vi "extract_calibration_standard_point_locations_debug.vi"() -> ()   [LabVIEW 2019]
uses:
  ParametersGlobal.vi
  <vilib>/vision/NI_Vision_Development_Module.lvlib
panel:
  out "Particle Measurements (Pixels)":dbl[][](array[numeric]) format="%.2f"
  out "Camera Input":T1(plugin-control)
  in  "Calibration file in":string="C:\\Users\\Mochi\\Dropbox\\LeiferShaevitz\\Github\\ProjectAPI\\LabviewVIs\\BoxA-PC_projector_to_camera_distortion.png"
  out "error out":errorcluster
  in  "error in (no error)":errorcluster
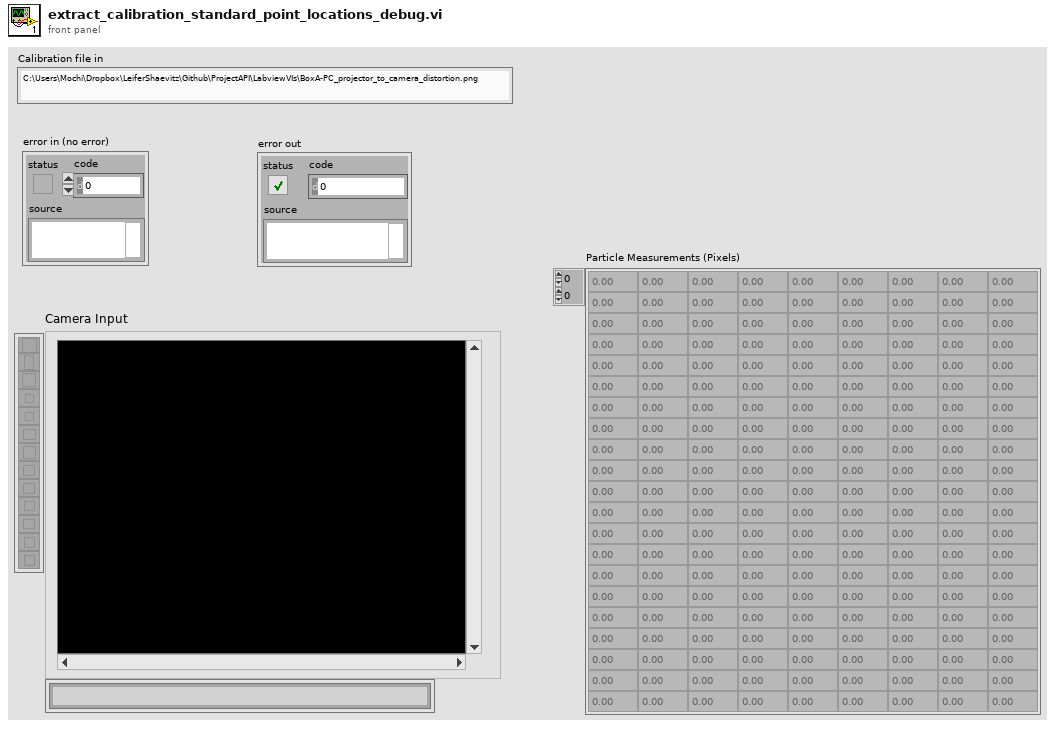
[diagram p1: front panel]
types:
  T1 = typedef "IMAQ Image.ctl" = refnum<image>
  T2 = typedef "Image Type" = u32
  T3 = cluster{"Left":i32, "Top":i32, "Right":i32, "Bottom":i32}
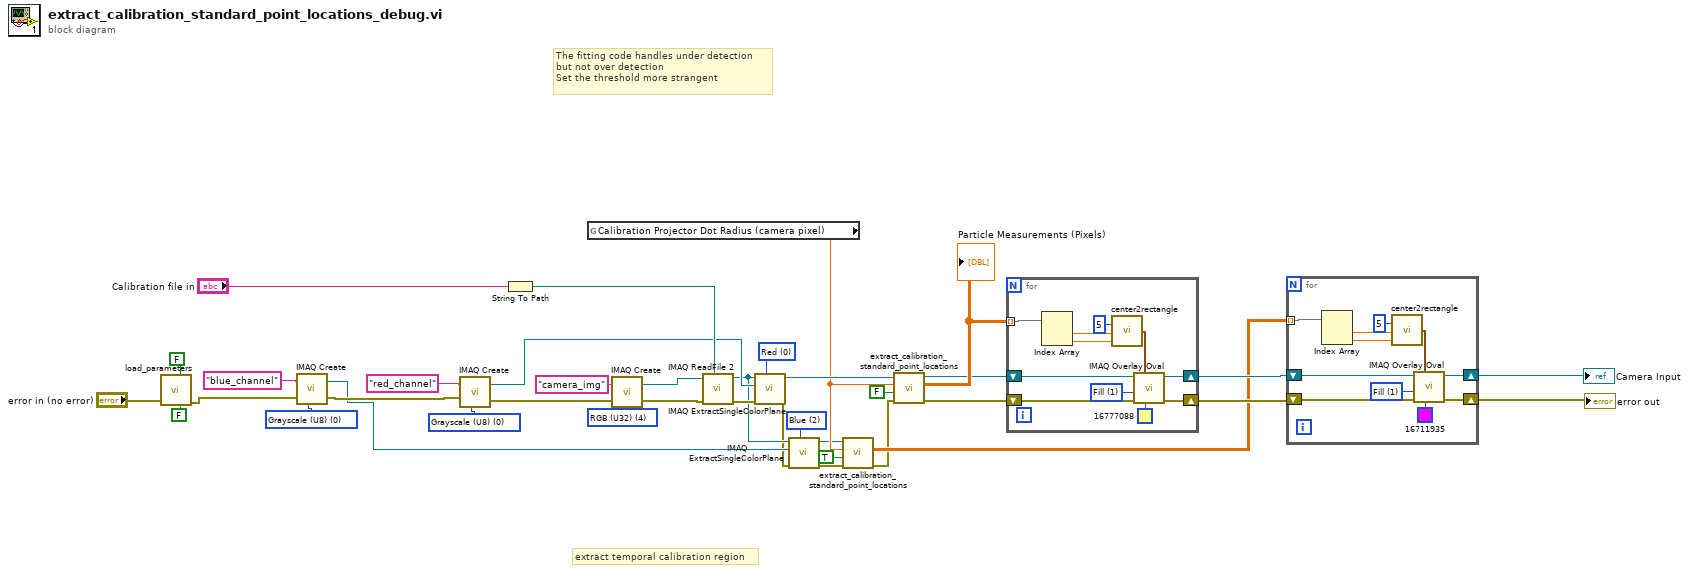
[diagram p0: block diagram]
diagram:
  w17 = 2 items=["Red", "Green", "Blue", "Hue", "Saturation", "Luminance", "Value", "Intensity"] ("Color Plane")
  w20 = T2 0 items=["Grayscale (U8)", "Grayscale (I16)", "Grayscale (SGL)", "Complex (CSG)", "RGB (U32)", "HSL (U32)", "RGB (U64)", "Grayscale (U16)"] ("Image Type")
  w24 = 0 items=["Red", "Green", "Blue", "Hue", "Saturation", "Luminance", "Value", "Intensity"] ("Color Plane")
  w31 = T2 0 items=["Grayscale (U8)", "Grayscale (I16)", "Grayscale (SGL)", "Complex (CSG)", "RGB (U32)", "HSL (U32)", "RGB (U64)", "Grayscale (U16)"] ("Image Type")
  w34 = T2 4 items=["Grayscale (U8)", "Grayscale (I16)", "Grayscale (SGL)", "Complex (CSG)", "RGB (U32)", "HSL (U32)", "RGB (U64)", "Grayscale (U16)"] ("Image Type")
  # "The fitting code handles under detection\nbut not over detection\nSet the threshold more strangent"
  # "extract temporal calibration region"
  n1 = call "load_parameters.vi"("Create Data Folder (T)"=FALSE, "Set Up Projector and Camera (T)"=FALSE, "error in (no error)"="error in (no error)") -> ("error out"=w19:errorcluster)  [unwired: 6 in, 2 out]
  n2 = call "IMAQ Create"("Image Name"="blue_channel", "Image Type"=w20, "error in (no error)"=w19) -> ("New Image"=w16:T1, "error out"=w18:errorcluster)  [unwired: 2 in]
  n3 = call "IMAQ Create"("Image Name"="red_channel", "Image Type"=w31, "error in (no error)"=w18) -> ("New Image"=w22:T1, "error out"=w28:errorcluster)  [unwired: 2 in]
  n4 = String To Path(string="Calibration file in") -> (path=w25:path)
  n5 = global read "ParametersGlobal.vi" "Calibration Projector Dot Radius (camera pixel)"() -> (w14:dbl)
  n6 = call "IMAQ Create"("Image Name"="camera_img", "Image Type"=w34, "error in (no error)"=w28) -> ("New Image"=w27:T1, "error out"=w30:errorcluster)  [unwired: 2 in]
  n7 = call "IMAQ ReadFile 2"("File Path"=w25, "error in (no error)"=w30, "Image"=w27) -> ("error out"=w29:errorcluster, "Image Out"=w15:T1)  [unwired: 4 in, 3 out]
  n8 = call "IMAQ ExtractSingleColorPlane"("Color Plane"=w24, "error in (no error)"=w29, "Image Dst"=w22, "Image Src"=w15) -> ("error out"=w3:errorcluster, "Image Dst Out"=w23:T1)  [unwired: 6 in]
  n9 = call "IMAQ ExtractSingleColorPlane"("Color Plane"=w17, "error in (no error)"=w3, "Image Dst"=w16, "Image Src"=w15) -> ("error out"=w12:errorcluster, "Image Dst Out"=w13:T1)  [unwired: 6 in]
  n10 = call "extract_calibration_standard_point_locations.vi"("error in (no error)"=w12, "Agar (T) Paper (F)"=TRUE, "expected dot radius (camera pixels)"=w14, "Image Src"=w13) -> ("error out"=w2:errorcluster, "Particle Measurements (Pixels)"=w9:dbl[][])  [unwired: 5 in, 1 out]
  n11 = call "extract_calibration_standard_point_locations.vi"("error in (no error)"=w2, "Agar (T) Paper (F)"=FALSE, "expected dot radius (camera pixels)"=w14, "Image Src"=w23) -> ("error out"=w1:errorcluster, "Particle Measurements (Pixels)"=w26:dbl[][], "Image Out (duplicate)"=w6:T1)  [unwired: 5 in]
  "Particle Measurements (Pixels)" <- w26
  n12 = for {
    shift-right: [w45] -> w11
    shift-left: w1 -> [w48]
    shift-right: [w46] -> w10
    shift-left: w6 -> [w47]
    tunnel: w26 -> [w42] mode=indexing
    w49 = u32 1 items=["Frame", "Fill"] ("Drawing Mode (Frame)")
    n13 = Index Array(array=w42) -> (element #1=w40:dbl, element #2=w39:dbl)  [unwired: 2 in]
    n14 = call "center2rectangle.vi"("Center Y"=w39, "Center X"=w40, "Box Half Size"=5) -> ("Box Rectangle"=w41:T3)
    n15 = call "IMAQ Overlay Oval"("Color"=u32 16777088, "error in (no error)"=w48, "Drawing Mode (Frame)"=w49, "Bounding Rectangle"=w41, "Image"=w47) -> ("error out"=w45:errorcluster, "Image Out"=w46:T1)  [unwired: 5 in]
  }
  n16 = for {
    shift-right: [w56] -> w7
    shift-left: w11 -> [w59]
    shift-right: [w57] -> w8
    shift-left: w10 -> [w58]
    tunnel: w9 -> [w53] mode=indexing
    w60 = u32 1 items=["Frame", "Fill"] ("Drawing Mode (Frame)")
    n17 = Index Array(array=w53) -> (element #1=w51:dbl, element #2=w50:dbl)  [unwired: 2 in]
    n18 = call "center2rectangle.vi"("Center Y"=w50, "Center X"=w51, "Box Half Size"=5) -> ("Box Rectangle"=w52:T3)
    n19 = call "IMAQ Overlay Oval"("Color"=u32 16711935, "error in (no error)"=w59, "Drawing Mode (Frame)"=w60, "Bounding Rectangle"=w52, "Image"=w58) -> ("error out"=w56:errorcluster, "Image Out"=w57:T1)  [unwired: 5 in]
  }
  "error out" <- w7
  "Camera Input" <- w8
